vi "Timing Sort by Priority.vi"() -> ()   [LabVIEW 2017]
uses:
  Source/Engine/Classes/Transfer/DSF.Engine.Transfer.lvclass
  Source/Shared/Typedefs/DSF.Shared.Typedefs.Direction.ctl
  Source/Shared/Classes/Timing/DSF.Shared.Timing.lvclass/DSF.Shared.Timing.ctl
  Source/Engine/Classes/Transfer/DSF.Engine.Transfer Group.lvclass/DSF.Engine.Transfer Group.ctl
  Source/Shared/Classes/Timing/DSF.Shared.Timing.lvclass
  Source/Engine/Classes/Transfer/DSF.Engine.Transfer Group.lvclass
  Source/DSF.Shared.lvlib
panel:
  out "group post-sort":u64[](array[numeric])
  out "post-sort":u64[](array[numeric])
  out "pre-sort":u64[](array[numeric])
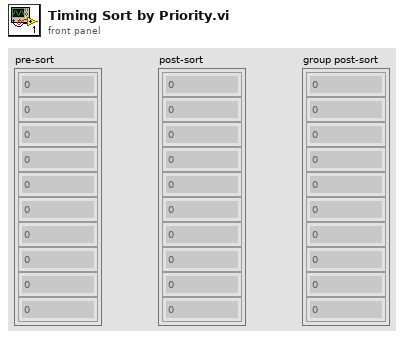
[diagram p1: front panel]
types:
  T1 = typedef "DSF.Shared.lvlib/DSF.Shared.Typedefs.Direction.ctl" = enum8{"Tx", "Rx"}
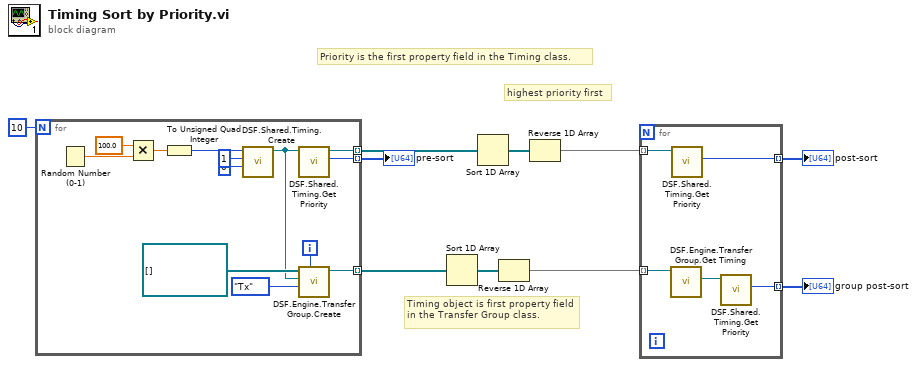
[diagram p0: block diagram]
diagram:
  # "Timing object is first property field in the Transfer Group class."
  # "highest priority first"
  # "Priority is the first property field in the Timing class."
  n1 = for {
    N: 10 -> [_]
    tunnel: [w17] -> w9 mode=indexing
    tunnel: [w16] -> w8 mode=indexing
    tunnel: [w11] -> w3 mode=indexing
    i -> [w15]
    n2 = Random Number (0-1)() -> (number: 0 to 1=w23:dbl)
    n3 = Multiply(x=100.0, y=w23) -> (x*y=w21:dbl)
    n4 = To Unsigned Quad Integer(1:w21) -> (0:w20:u64)
    n5 = call "DSF.Shared.Timing.Create.vi"("Offset"=u64 0, "Decimation"=u64 1, "Priority"=w20) -> ("Timing"=w12:refnum<class "DSF.Shared.Timing.lvclass">)  [unwired: 7 in, 1 out]
    n6 = call "DSF.Shared.Timing.Get Priority.vi"("Timing in"=w12) -> ("Priority"=w16:u64, "Timing out"=w17:refnum<class "DSF.Shared.Timing.lvclass">)  [unwired: 9 in]
    n7 = call "DSF.Engine.Transfer Group.Create.vi"("id"=w15, "Direction"=DSF.Shared.Typedefs.Direction."Tx", "Timing"=w12, "Transfers"=refnum<class "DSF.Engine.Transfer.lvclass">[] []) -> ("Transfer Group out"=w11:refnum<class "DSF.Engine.Transfer Group.lvclass">)  [unwired: 6 in, 1 out]
  }
  "pre-sort" <- w8
  n8 = Sort 1D Array(array=w3) -> (sorted array=w4:refnum<class "DSF.Engine.Transfer Group.lvclass">[])
  n9 = Sort 1D Array(array=w9) -> (sorted array=w6:refnum<class "DSF.Shared.Timing.lvclass">[])
  n10 = Reverse 1D Array(array=w4) -> (reversed array=w2:refnum<class "DSF.Engine.Transfer Group.lvclass">[])
  n11 = Reverse 1D Array(array=w6) -> (reversed array=w5:refnum<class "DSF.Shared.Timing.lvclass">[])
  n12 = for {
    tunnel: w5 -> [w28] mode=indexing
    tunnel: [w27] -> w7 mode=indexing
    tunnel: w2 -> [w26] mode=indexing
    tunnel: [w24] -> w1 mode=indexing
    n13 = call "DSF.Engine.Transfer Group.Get Timing.vi"("Transfer Group in"=w26) -> ("Timing"=w25:refnum<class "DSF.Shared.Timing.lvclass">)  [unwired: 9 in, 1 out]
    n14 = call "DSF.Shared.Timing.Get Priority.vi"("Timing in"=w28) -> ("Priority"=w27:u64)  [unwired: 9 in, 1 out]
    n15 = call "DSF.Shared.Timing.Get Priority.vi"("Timing in"=w25) -> ("Priority"=w24:u64)  [unwired: 9 in, 1 out]
  }
  "post-sort" <- w7
  "group post-sort" <- w1
